vi "scope_test.vi"() -> ()   [LabVIEW 2021]
panel:
  in  "CH1 Coupling":u16(ring) items=["AC", "DC", "GND"]
  in  "Stop button":bool
  in  "End program":bool
  in  "stop":bool
  in  "OK Button":bool
  in  "Trigger Value":dbl
  in  "Trigger Level":dbl
  in  "Horizontal Positon":dbl(knob) scale=0.002..5.0
  in  "Horizontal Scale":dbl(knob) scale=0.002..5.0
  in  "Numeric 2":dbl
  in  "Numeric":dbl
  in  "CH2 Volts/DIV":dbl(knob) scale=0.002..5.0
  in  "CH1 Volts/DIV":dbl(knob) scale=0.002..5.0
  in  "VISA name":refnum<visa-resource-name>
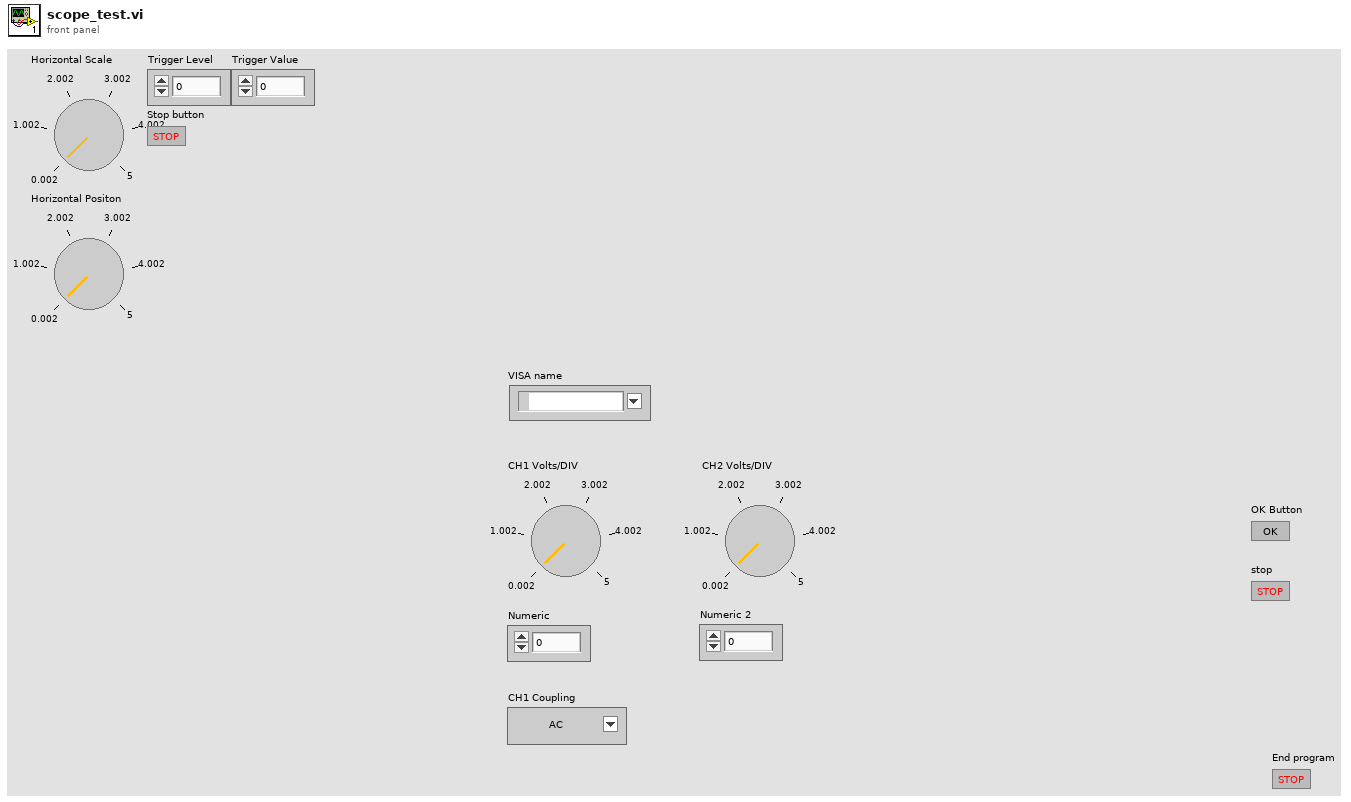
[diagram p1: front panel]
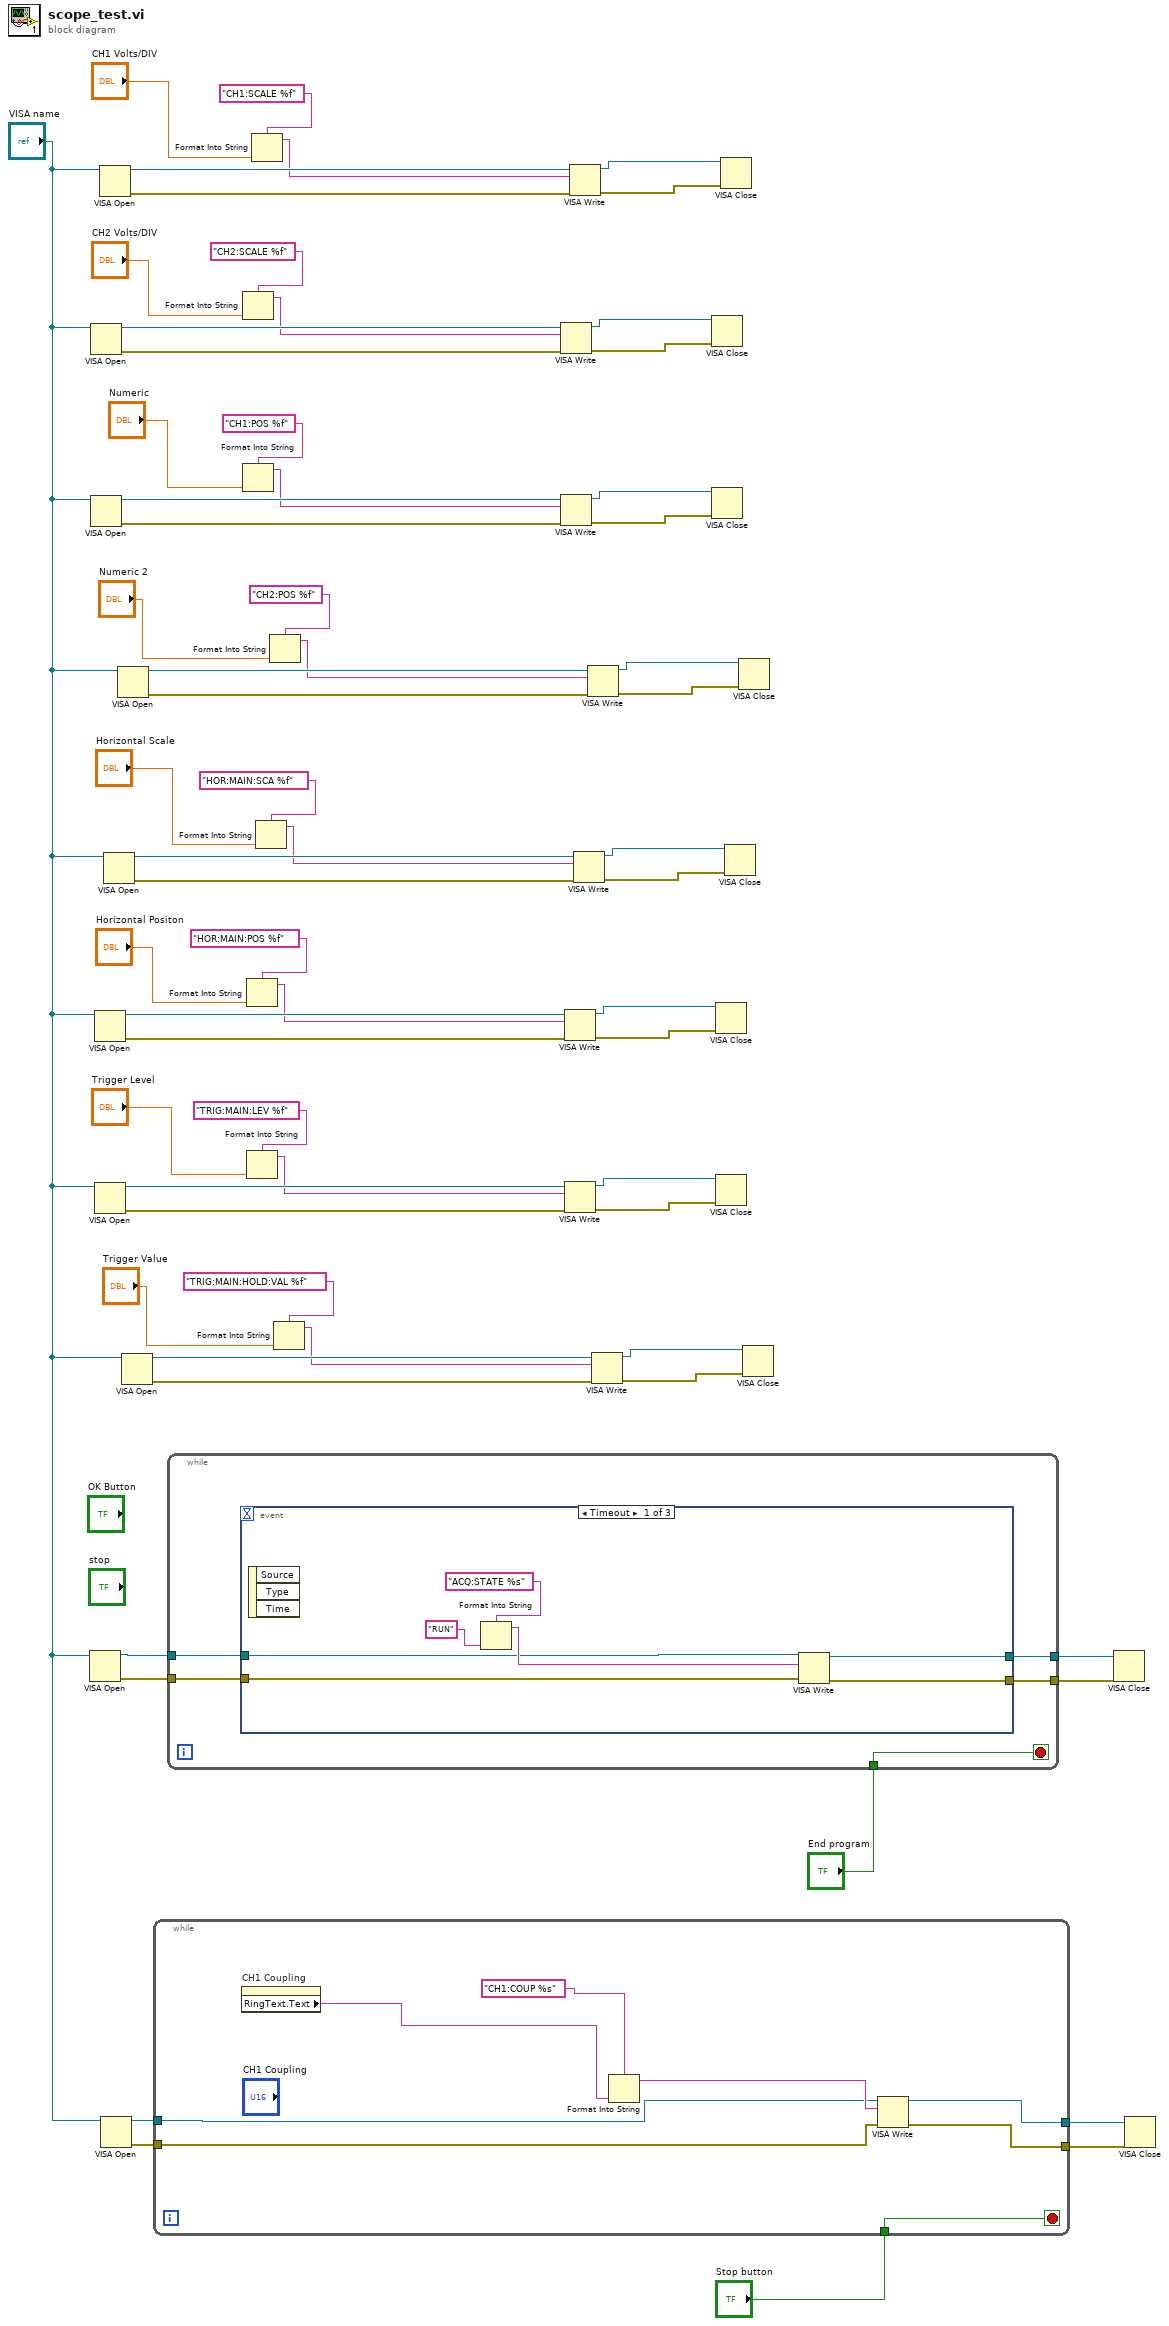
[diagram p0: block diagram]
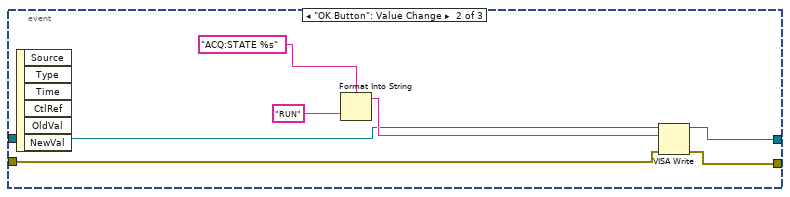
[diagram p2: hidden frame]
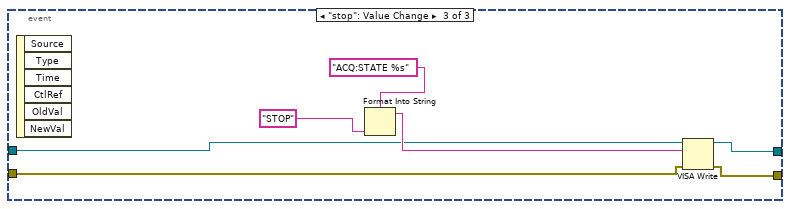
[diagram p3: hidden frame]
diagram:
  n1 = VISA Open(VISA resource name="VISA name") -> (VISA resource name=w9:refnum<visa-resource-name>, error out=w10:errorcluster)  [unwired: 4 in]
  n2 = VISA Open(VISA resource name="VISA name") -> (VISA resource name=w60:refnum<visa-resource-name>, error out=w61:errorcluster)  [unwired: 4 in]
  n3 = VISA Open(VISA resource name="VISA name") -> (VISA resource name=w54:refnum<visa-resource-name>, error out=w55:errorcluster)  [unwired: 4 in]
  n4 = VISA Open(VISA resource name="VISA name") -> (VISA resource name=w32:refnum<visa-resource-name>, error out=w33:errorcluster)  [unwired: 4 in]
  n5 = VISA Open(VISA resource name="VISA name") -> (VISA resource name=w26:refnum<visa-resource-name>, error out=w27:errorcluster)  [unwired: 4 in]
  n6 = VISA Open(VISA resource name="VISA name") -> (VISA resource name=w66:refnum<visa-resource-name>, error out=w67:errorcluster)  [unwired: 4 in]
  n7 = VISA Open(VISA resource name="VISA name") -> (VISA resource name=w5:refnum<visa-resource-name>, error out=w6:errorcluster)  [unwired: 4 in]
  n8 = VISA Open(VISA resource name="VISA name") -> (VISA resource name=w38:refnum<visa-resource-name>, error out=w39:errorcluster)  [unwired: 4 in]
  n9 = VISA Open(VISA resource name="VISA name") -> (VISA resource name=w48:refnum<visa-resource-name>, error out=w49:errorcluster)  [unwired: 4 in]
  n10 = VISA Open(VISA resource name="VISA name") -> (VISA resource name=w20:refnum<visa-resource-name>, error out=w21:errorcluster)  [unwired: 4 in]
  n11 = while {
    tunnel: "Stop button" -> [w75]
    tunnel: w6 -> [w70]
    tunnel: w5 -> [w68]
    tunnel: [w74] -> w4
    tunnel: [w73] -> w3
    stop <- w75 stop-if-true
    n12 = property on="CH1 Coupling" class="Ring (strict)"() -> ("RingText.Text"=w72:string)  [unwired: 2 in, 2 out]
    n13 = Format Into String(format string="CH1:COUP %s", w72) -> (resulting string=w69:string)  [unwired: 2 in, 1 out]
    n14 = VISA Write(VISA resource name=w68, write buffer=w69, error in (no error)=w70) -> (VISA resource name out=w73:refnum<visa-resource-name>, error out=w74:errorcluster)  [unwired: 1 out]
  }
  n15 = while {
    tunnel: "End program" -> [w80]
    tunnel: w10 -> [w79]
    tunnel: w9 -> [w78]
    tunnel: [w77] -> w8
    tunnel: [w76] -> w7
    stop <- w80 stop-if-true
    n16 = event shown="[0] Timeout" {
      selector: _ -> [_ _ _]
      dyn-events: _ -> [_ _ _]
      timeout: _ -> [_ _ _]
      tunnel: w79 -> [w85 w91 w98]
      tunnel: w78 -> [w84 w92 w99]
      tunnel: [w83 w90 w96] -> w77
      tunnel: [w82 w89 w97] -> w76
      event Timeout {
        n17 = event-data() -> ()  [unwired: 1 in, 3 out]
        n18 = Format Into String(format string="ACQ:STATE %s", "RUN" ("input 1")) -> (resulting string=w87:string)  [unwired: 2 in, 1 out]
        n19 = VISA Write(VISA resource name=w84, write buffer=w87, error in (no error)=w85) -> (VISA resource name out=w82:refnum<visa-resource-name>, error out=w83:errorcluster)  [unwired: 1 out]
      }
      event "OK Button": Value Change {
        n20 = event-data() -> ()  [unwired: 1 in, 6 out]
        n21 = Format Into String(format string="ACQ:STATE %s", "RUN") -> (resulting string=w94:string)  [unwired: 2 in, 1 out]
        n22 = VISA Write(VISA resource name=w92, write buffer=w94, error in (no error)=w91) -> (VISA resource name out=w89:refnum<visa-resource-name>, error out=w90:errorcluster)  [unwired: 1 out]
      }
      event "stop": Value Change {
        n23 = event-data() -> ()  [unwired: 1 in, 6 out]
        n24 = Format Into String(format string="ACQ:STATE %s", "STOP") -> (resulting string=w101:string)  [unwired: 2 in, 1 out]
        n25 = VISA Write(VISA resource name=w99, write buffer=w101, error in (no error)=w98) -> (VISA resource name out=w97:refnum<visa-resource-name>, error out=w96:errorcluster)  [unwired: 1 out]
      }
    }
  }
  n26 = Format Into String(format string="CH2:SCALE %f", "CH2 Volts/DIV") -> (resulting string=w56:string)  [unwired: 2 in, 1 out]
  n27 = Format Into String(format string="CH1:POS %f", "Numeric") -> (resulting string=w50:string)  [unwired: 2 in, 1 out]
  n28 = Format Into String(format string="HOR:MAIN:POS %f", "Horizontal Positon") -> (resulting string=w28:string)  [unwired: 2 in, 1 out]
  n29 = Format Into String(format string="TRIG:MAIN:LEV %f", "Trigger Level") -> (resulting string=w22:string)  [unwired: 2 in, 1 out]
  n30 = Format Into String(format string="CH1:SCALE %f", "CH1 Volts/DIV") -> (resulting string=w62:string)  [unwired: 2 in, 1 out]
  n31 = Format Into String(format string="HOR:MAIN:SCA %f", "Horizontal Scale") -> (resulting string=w34:string)  [unwired: 2 in, 1 out]
  n32 = Format Into String(format string="CH2:POS %f", "Numeric 2") -> (resulting string=w44:string)  [unwired: 2 in, 1 out]
  n33 = Format Into String(format string="TRIG:MAIN:HOLD:VAL %f", "Trigger Value") -> (resulting string=w16:string)  [unwired: 2 in, 1 out]
  n34 = VISA Write(VISA resource name=w60, write buffer=w56, error in (no error)=w61) -> (VISA resource name out=w57:refnum<visa-resource-name>, error out=w58:errorcluster)  [unwired: 1 out]
  n35 = VISA Write(VISA resource name=w54, write buffer=w50, error in (no error)=w55) -> (VISA resource name out=w51:refnum<visa-resource-name>, error out=w52:errorcluster)  [unwired: 1 out]
  n36 = VISA Write(VISA resource name=w32, write buffer=w28, error in (no error)=w33) -> (VISA resource name out=w29:refnum<visa-resource-name>, error out=w30:errorcluster)  [unwired: 1 out]
  n37 = VISA Write(VISA resource name=w26, write buffer=w22, error in (no error)=w27) -> (VISA resource name out=w23:refnum<visa-resource-name>, error out=w24:errorcluster)  [unwired: 1 out]
  n38 = VISA Write(VISA resource name=w66, write buffer=w62, error in (no error)=w67) -> (VISA resource name out=w63:refnum<visa-resource-name>, error out=w64:errorcluster)  [unwired: 1 out]
  n39 = VISA Write(VISA resource name=w38, write buffer=w34, error in (no error)=w39) -> (VISA resource name out=w35:refnum<visa-resource-name>, error out=w36:errorcluster)  [unwired: 1 out]
  n40 = VISA Write(VISA resource name=w48, write buffer=w44, error in (no error)=w49) -> (VISA resource name out=w45:refnum<visa-resource-name>, error out=w46:errorcluster)  [unwired: 1 out]
  n41 = VISA Write(VISA resource name=w20, write buffer=w16, error in (no error)=w21) -> (VISA resource name out=w17:refnum<visa-resource-name>, error out=w18:errorcluster)  [unwired: 1 out]
  n42 = VISA Close(VISA resource name=w57, error in (no error)=w58) -> ()  [unwired: 1 out]
  n43 = VISA Close(VISA resource name=w51, error in (no error)=w52) -> ()  [unwired: 1 out]
  n44 = VISA Close(VISA resource name=w29, error in (no error)=w30) -> ()  [unwired: 1 out]
  n45 = VISA Close(VISA resource name=w23, error in (no error)=w24) -> ()  [unwired: 1 out]
  n46 = VISA Close(VISA resource name=w63, error in (no error)=w64) -> ()  [unwired: 1 out]
  n47 = VISA Close(VISA resource name=w35, error in (no error)=w36) -> ()  [unwired: 1 out]
  n48 = VISA Close(VISA resource name=w45, error in (no error)=w46) -> ()  [unwired: 1 out]
  n49 = VISA Close(VISA resource name=w17, error in (no error)=w18) -> ()  [unwired: 1 out]
  n50 = VISA Close(VISA resource name=w7, error in (no error)=w8) -> ()  [unwired: 1 out]
  n51 = VISA Close(VISA resource name=w3, error in (no error)=w4) -> ()  [unwired: 1 out]
